vi "SQL_test_template_data_insert.vi"(10 "表格控件":string[][](table), 11 "tempNo":string) -> (3 "error out":errorcluster)   [LabVIEW 2014]
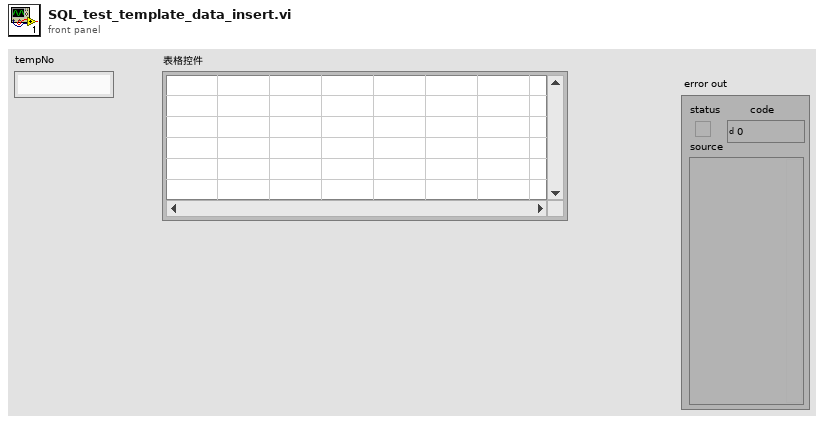
[diagram p1: front panel]
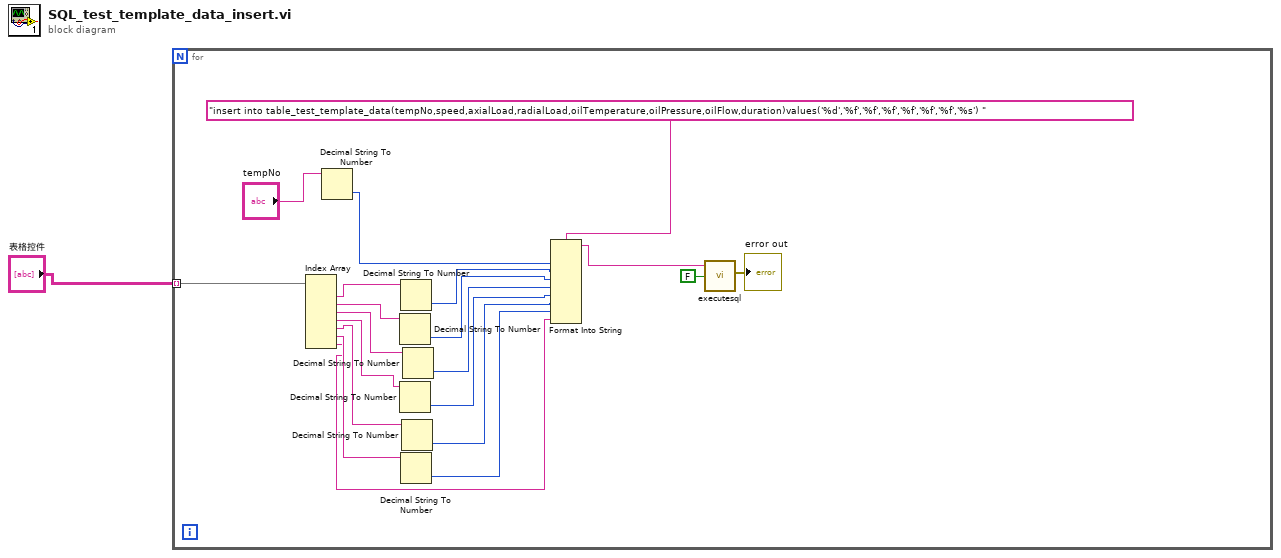
[diagram p0: block diagram]
diagram:
  n1 = for {
    tunnel: "表格控件" -> [w20] mode=indexing
    n2 = Index Array(array=w20) -> (element #1=w19:string, element #2=w18:string, element #3=w16:string, element #4=w14:string, element #5=w12:string, element #6=w10:string, element #7=w8:string)  [unwired: 7 in]
    n3 = Decimal String To Number(string="tempNo") -> (number=w2:i32)  [unwired: 2 in, 1 out]
    n4 = Decimal String To Number(string=w18) -> (number=w17:i32)  [unwired: 2 in, 1 out]
    n5 = Decimal String To Number(string=w14) -> (number=w13:i32)  [unwired: 2 in, 1 out]
    n6 = Decimal String To Number(string=w19) -> (number=w3:i32)  [unwired: 2 in, 1 out]
    n7 = Decimal String To Number(string=w10) -> (number=w9:i32)  [unwired: 2 in, 1 out]
    n8 = Decimal String To Number(string=w12) -> (number=w11:i32)  [unwired: 2 in, 1 out]
    n9 = Decimal String To Number(string=w16) -> (number=w15:i32)  [unwired: 2 in, 1 out]
    n10 = Format Into String(format string="insert into table_test_template_data(tempNo,speed,axialLoad,radialLoad,oilTemperature,oilPressure,oilFlow,duration)values('%d','%f','%f','%f','%f','%f','%f','%s') ", w2, w3, w17, w15, w13, w11, w9, w8) -> (resulting string=w7:string)  [unwired: 2 in, 1 out]
    n11 = call "executesql.vi"("Return Data (T)"=FALSE, "Command Text"=w7) -> ("error out"=→"error out":errorcluster)  [unwired: 5 in, 1 out]
  }
